vi "9.1 Case Structures.vi"() -> ()   [LabVIEW 2019]
panel:
  out "Message 3":string
  out "Result":dbl
  in  "Y":dbl
  in  "X":dbl
  in  "operation":T1(ring)
  in  "error control":errorcluster
  out "Message 2":string
  in  "Current temperature 2":dbl
  out "Message":string
  in  "Threshold temperature":dbl
  in  "Current temperature":dbl
  # "BOOLEAN CASE"
  # "NUMERIC CASE"
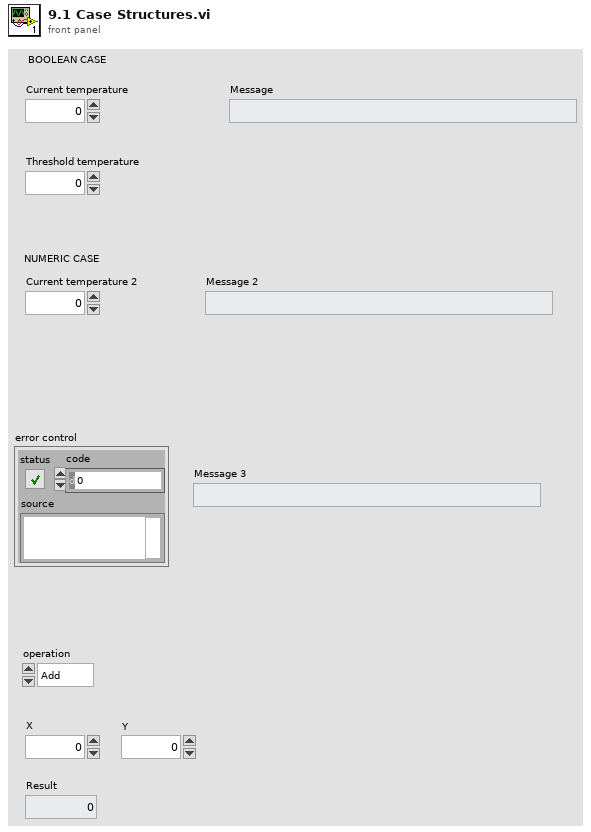
[diagram p1: front panel]
types:
  T1 = enum16{"Add", "Subtract", "Multiply", "Divide", "Remainder"}
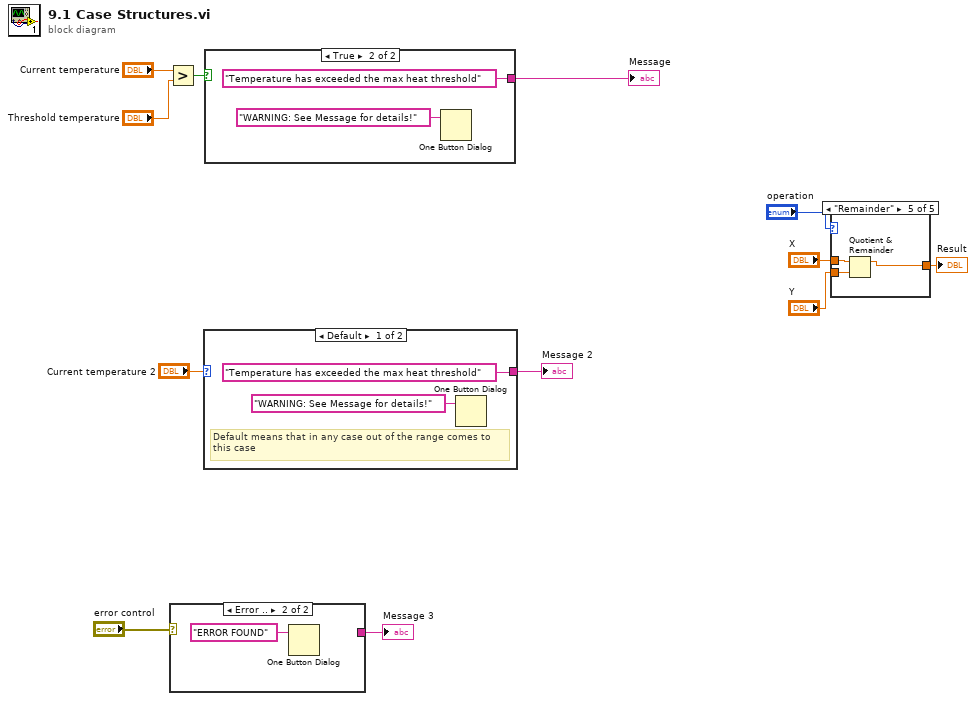
[diagram p0: block diagram]
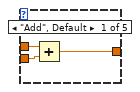
[diagram p2: hidden frame]
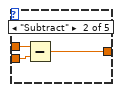
[diagram p3: hidden frame]
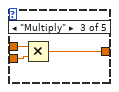
[diagram p4: hidden frame]
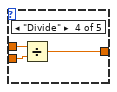
[diagram p5: hidden frame]
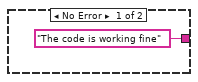
[diagram p6: hidden frame]
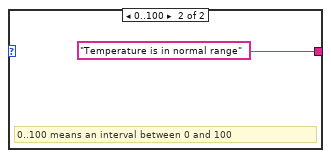
[diagram p7: hidden frame]
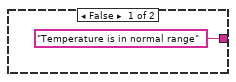
[diagram p8: hidden frame]
diagram:
  n1 = Greater?(x="Current temperature", y="Threshold temperature") -> (0:w10:bool)
  n2 = case shown="Error .." "error control" {
    tunnel: ["The code is working fine" _] -> w1
    frame No Error {
    }
    frame Error {
      n3 = One Button Dialog(message="ERROR FOUND") -> ()  [unwired: 1 in, 1 out]
    }
  }
  "Message 3" <- w1
  n4 = case shown="Default" "Current temperature 2" {
    tunnel: ["Temperature has exceeded the max heat threshold" "Temperature is in normal range"] -> w7
    frame Default {
      # "Default means that in any case out of the range comes to this case"
      n5 = One Button Dialog(message="WARNING: See Message for details!") -> ()  [unwired: 1 in, 1 out]
    }
    frame 0..100 {
      # "0..100 means an interval between 0 and 100"
    }
  }
  "Message 2" <- w7
  n6 = case shown="True" w10 {
    tunnel: ["Temperature is in normal range" "Temperature has exceeded the max heat threshold"] -> w9
    frame False {
    }
    frame True {
      n7 = One Button Dialog(message="WARNING: See Message for details!") -> ()  [unwired: 1 in, 1 out]
    }
  }
  "Message" <- w9
  n8 = case shown="\"Remainder\"" "operation" {
    tunnel: "X" -> [w23 w26 w29 w31 w35]
    tunnel: "Y" -> [w22 w25 w28 w30 w34]
    tunnel: [w21 w24 w27 w32 w33] -> w2
    frame "Add", Default {
      n9 = Add(x=w23, y=w22) -> (x+y=w21:dbl)
    }
    frame "Subtract" {
      n10 = Subtract(x=w26, y=w25) -> (x-y=w24:dbl)
    }
    frame "Multiply" {
      n11 = Multiply(x=w29, y=w28) -> (x*y=w27:dbl)
    }
    frame "Divide" {
      n12 = Divide(x=w31, y=w30) -> (x/y=w32:dbl)
    }
    frame "Remainder" {
      n13 = Quotient & Remainder(x=w35, y=w34) -> (x-y*floor(x/y)=w33:dbl)  [unwired: 1 out]
    }
  }
  "Result" <- w2
